vi "DMARS_Frame_v2_write_PXI.vi"(11 "DMARS":dbl[](array[numeric])) -> (0 "No DMARS string":bool, 3 "string_Out":string)   [LabVIEW 2017]
panel:
  out "unsigned 32bit integer":u32
  out "SubFrame":u8
  out "sec":dbl
  out "size(s)":i32
  out "output array":u8[](array[numeric]) format="%x"
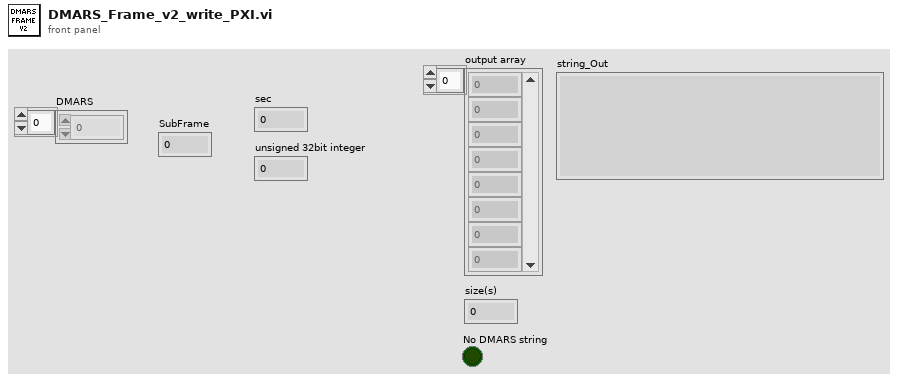
[diagram p1: front panel]
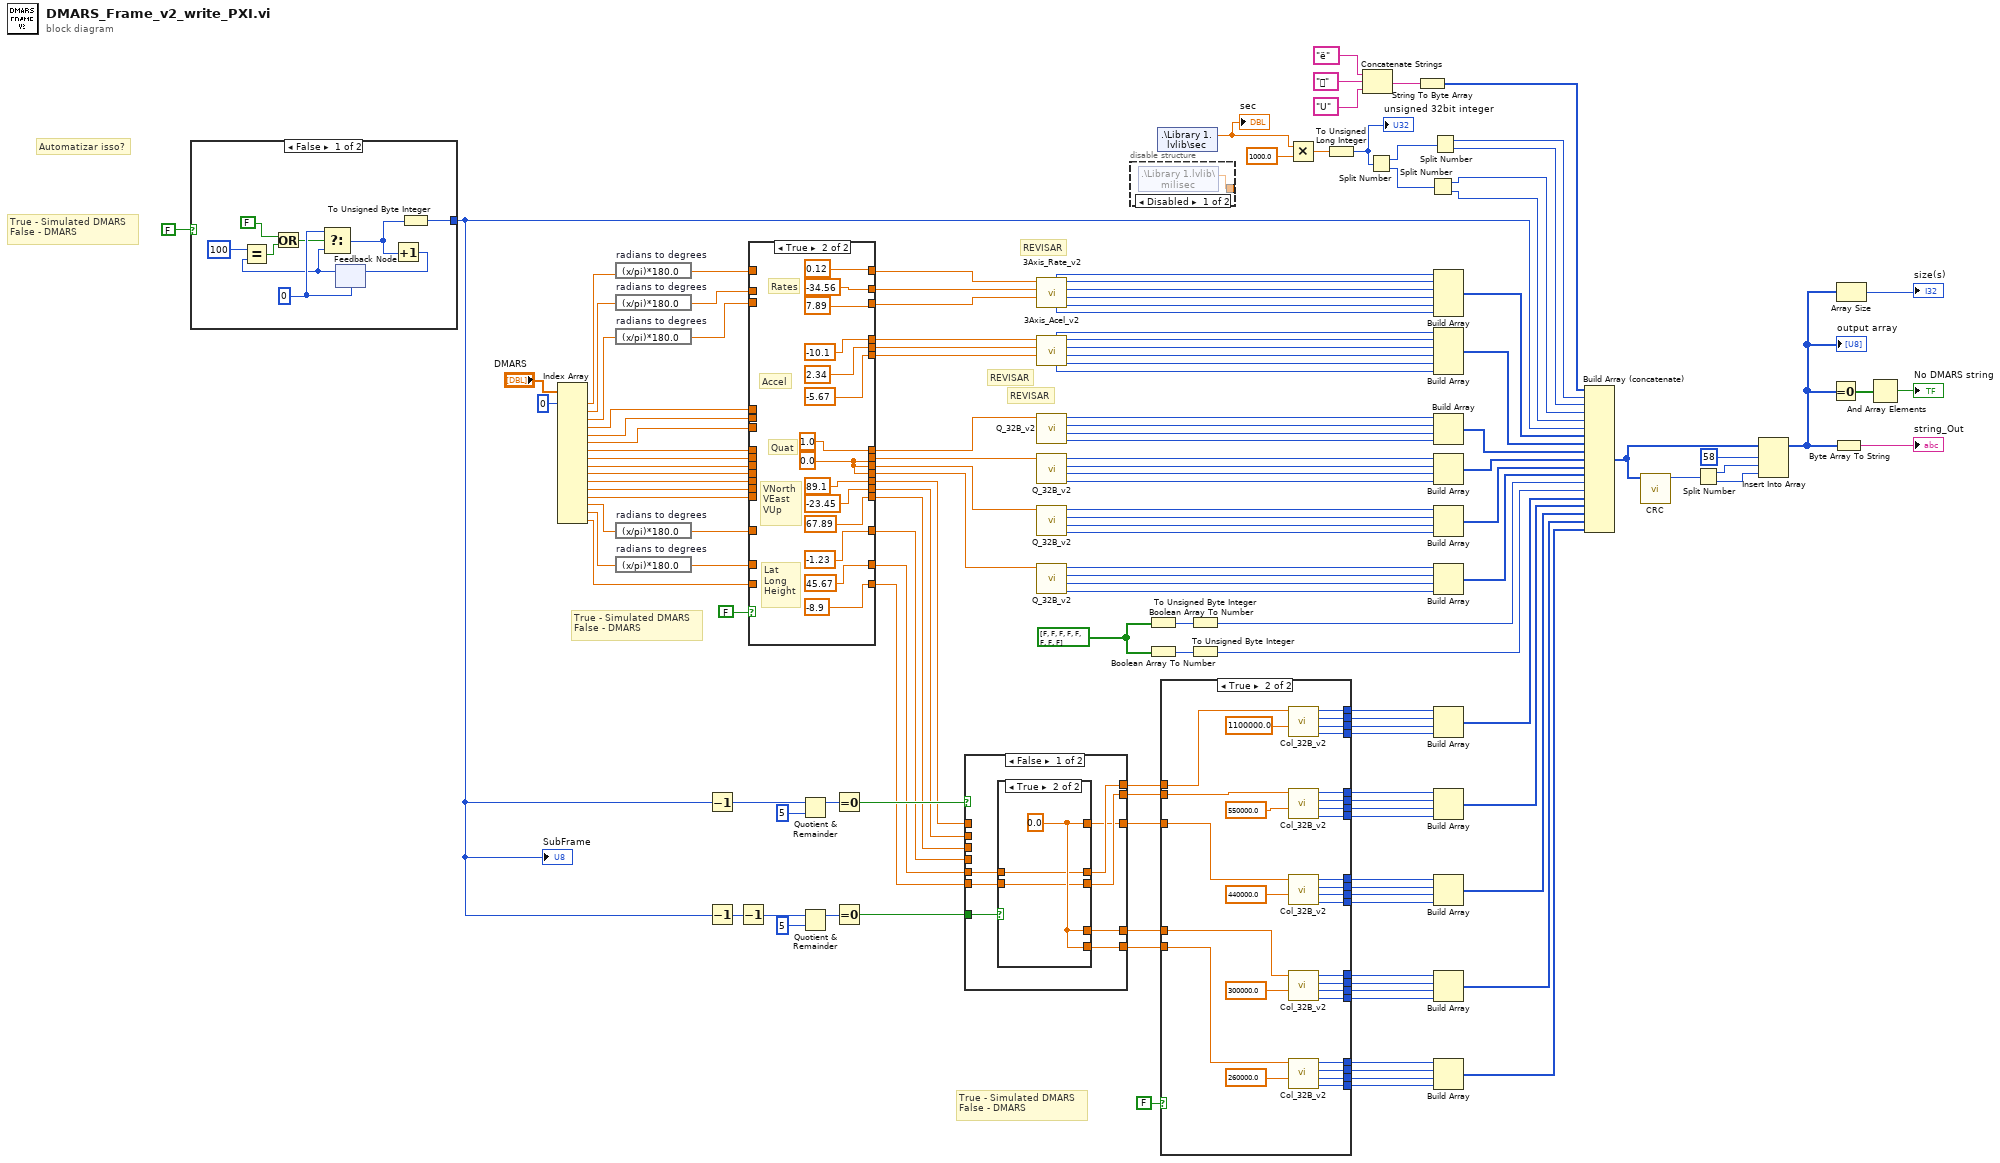
[diagram p0: block diagram]
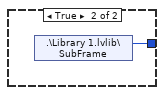
[diagram p2: hidden frame]
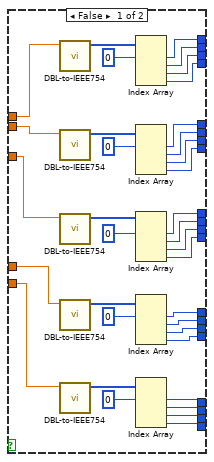
[diagram p5: hidden frame]
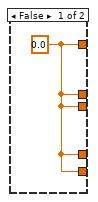
[diagram p6: hidden frame]
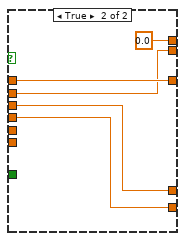
[diagram p7: hidden frame]
diagram:
  w130 = bool[] [FALSE, FALSE, FALSE, FALSE, FALSE, FALSE, FALSE, FALSE] ("Byte 36")
  # "REVISAR"
  # "REVISAR"
  # "REVISAR"
  # "True - Simulated DMARS\nFalse - DMARS"
  # "True - Simulated DMARS\nFalse - DMARS"
  # "Automatizar isso?"
  # "True - Simulated DMARS\nFalse - DMARS"
  n1 = case shown="False" FALSE {
    tunnel: [w148 w156] -> w120
    frame False {
      w155 = 0 ("x")
      n2 = feedback #1(w155) -> (w150:i32)
      n3 = Equal?(x=100, y=w150) -> (x = y?=w151:bool)
      n4 = Or(x=FALSE, y=w151) -> (x .or. y?=w152:bool)
      n5 = Select(t=w155, s=w152, f=w150) -> (s? t:f=w153:i32)
      n6 = Increment(x=w153) -> (x+1=w154:i32)
      n7 = feedback-in #1(w154) -> ()
      n8 = To Unsigned Byte Integer(number=w153) -> (unsigned 8bit integer=w148:u8)
    }
    frame True {
      n9 = shared-variable ".\\Library 1.lvlib\\SubFrame"() -> (w156:u8)  [unwired: 1 in, 1 out]
    }
  }
  "SubFrame" <- w120
  n10 = Index Array(array="DMARS", index #1=0 ("index")) -> (element #1=w79:dbl, element #2=w77:dbl, element #3=w76:dbl, element #4=w105:dbl, element #5=w103:dbl, element #6=w101:dbl, element #7=w99:dbl, element #8=w97:dbl, element #9=w96:dbl, element #10=w93:dbl, element #11=w91:dbl, element #12=w89:dbl, element #13=w87:dbl, element #14=w113:dbl, element #15=w112:dbl, element #16=w81:dbl)  [unwired: 15 in]
  n11 = expression code="(x/pi)*180.0" "radians to degrees"(w79) -> (w78:dbl)
  n12 = expression code="(x/pi)*180.0" "radians to degrees"(w77) -> (w75:dbl)
  n13 = expression code="(x/pi)*180.0" "radians to degrees"(w76) -> (w74:dbl)
  n14 = expression code="(x/pi)*180.0" "radians to degrees"(w113) -> (w85:dbl)
  n15 = expression code="(x/pi)*180.0" "radians to degrees"(w112) -> (w83:dbl)
  n16 = Decrement(x=w120) -> (x-1=w125:u8)
  n17 = Decrement(x=w120) -> (x-1=w121:u8)
  n18 = Decrement(x=w121) -> (x-1=w124:u8)
  n19 = case shown="True" FALSE {
    tunnel: [w172 0.12 ("Numeric")] -> w109
    tunnel: w78 -> [w172 _]
    tunnel: [w171 -34.56 ("Numeric")] -> w108
    tunnel: w75 -> [w171 _]
    tunnel: [w157 7.89 ("Numeric")] -> w107
    tunnel: w74 -> [w157 _]
    tunnel: [w170 -10.1 ("Numeric")] -> w106
    tunnel: w105 -> [w170 _]
    tunnel: [w169 2.34 ("Numeric")] -> w104
    tunnel: w103 -> [w169 _]
    tunnel: [w168 -5.67 ("Numeric")] -> w102
    tunnel: w101 -> [w168 _]
    tunnel: [w167 1.0 ("Numeric")] -> w100
    tunnel: w99 -> [w167 _]
    tunnel: [w166 w179] -> w98
    tunnel: w97 -> [w166 _]
    tunnel: w96 -> [w165 _]
    tunnel: [w165 w179] -> w95
    tunnel: [w164 w179] -> w94
    tunnel: w93 -> [w164 _]
    tunnel: [w163 89.1 ("Numeric")] -> w92
    tunnel: w91 -> [w163 _]
    tunnel: [w162 -23.45 ("Numeric")] -> w90
    tunnel: w89 -> [w162 _]
    tunnel: [w161 67.89 ("Numeric")] -> w88
    tunnel: w87 -> [w161 _]
    tunnel: [w160 -1.23 ("Numeric")] -> w86
    tunnel: w85 -> [w160 _]
    tunnel: [w159 45.67 ("Numeric")] -> w84
    tunnel: w83 -> [w159 _]
    tunnel: [w158 -8.9 ("Numeric")] -> w82
    tunnel: w81 -> [w158 _]
    frame False {
    }
    frame True {
      w179 = 0.0 ("Numeric")
      # "Rates"
      # "Accel"
      # "Quat"
      # "VNorth\nVEast\nVUp"
      # "Lat\nLong\nHeight"
    }
  }
  n20 = Quotient & Remainder(x=w125, y=u8 5) -> (x-y*floor(x/y)=w127:u8)  [unwired: 1 out]
  n21 = Quotient & Remainder(x=w124, y=u8 5) -> (x-y*floor(x/y)=w123:u8)  [unwired: 1 out]
  n22 = Equal To 0?(x=w127) -> (x = 0?=w126:bool)
  n23 = Equal To 0?(x=w123) -> (x = 0?=w114:bool)
  n24 = case shown="False" w126 {
    tunnel: w92 -> [_ w202]
    tunnel: w90 -> [_ w201]
    tunnel: w88 -> [_ w200]
    tunnel: w86 -> [_ w199]
    tunnel: [w191 0.0] -> w119
    tunnel: [w189 w202] -> w118
    tunnel: [w190 w201] -> w117
    tunnel: [w188 w200] -> w116
    tunnel: [w187 w199] -> w115
    tunnel: w114 -> [w194 _]
    tunnel: w84 -> [w193 _]
    tunnel: w82 -> [w192 _]
    frame False {
      n25 = case shown="True" w194 {
        tunnel: w193 -> [_ w197]
        tunnel: w192 -> [_ w196]
        tunnel: [w195 w197] -> w191
        tunnel: [w195 w196] -> w190
        tunnel: [w195 w198] -> w189
        tunnel: [w195 w198] -> w188
        tunnel: [w195 w198] -> w187
        frame False {
          w195 = 0.0
        }
        frame True {
          w198 = 0.0
        }
      }
    }
    frame True {
    }
  }
  n26 = call "3Axis_Rate_v2.vi"("Roll_R"=w107, "Yaw_R"=w108, "Pitch_R"=w109) -> ("RRH"=w57:u8, "YRL"=w58:u8, "YRH"=w59:u8, "PRL"=w60:u8, "RRL"=w56:u8, "PRH"=w61:u8)  [unwired: 3 in]
  n27 = call "3Axis_Acel_v2.vi"("Roll_A"=w102, "Yaw_A"=w104, "Pitch_A"=w106) -> ("RAH"=w50:u8, "YAL"=w51:u8, "YAH"=w52:u8, "PAL"=w53:u8, "RAL"=w49:u8, "PAH"=w54:u8)  [unwired: 3 in]
  n28 = call "Q_32B_v2.vi"("Q_32B"=w100) -> ("LL"=w44:u8, "HL"=w45:u8, "LH"=w46:u8, "HH"=w47:u8)  [unwired: 7 in]
  n29 = call "Q_32B_v2.vi"("Q_32B"=w98) -> ("LL"=w39:u8, "HL"=w40:u8, "LH"=w41:u8, "HH"=w42:u8)  [unwired: 7 in]
  n30 = call "Q_32B_v2.vi"("Q_32B"=w95) -> ("LL"=w34:u8, "HL"=w35:u8, "LH"=w36:u8, "HH"=w37:u8)  [unwired: 7 in]
  n31 = call "Q_32B_v2.vi"("Q_32B"=w94) -> ("LL"=w29:u8, "HL"=w30:u8, "LH"=w31:u8, "HH"=w32:u8)  [unwired: 7 in]
  n32 = disable-structure shown="Disabled" {
    disable-tunnel: [w204 _] -> _
    frame Disabled {
      n33 = shared-variable ".\\Library 1.lvlib\\milisec"() -> (w204:dbl)  [unwired: 1 in, 1 out]
    }
    frame Enabled {
    }
  }
  n34 = Boolean Array To Number(Boolean array=w130) -> (number=w140:u32)
  n35 = Boolean Array To Number(Boolean array=w130) -> (number=w139:u32)
  n36 = shared-variable ".\\Library 1.lvlib\\sec"() -> (w63:dbl)  [unwired: 1 in, 1 out]
  "sec" <- w63
  n37 = case shown="True" FALSE {
    tunnel: [w208 w269] -> w5
    tunnel: [w205 w268] -> w2
    tunnel: [w206 w267] -> w3
    tunnel: [w207 w266] -> w4
    tunnel: [w209 w265] -> w7
    tunnel: [w210 w264] -> w8
    tunnel: [w211 w263] -> w9
    tunnel: [w212 w262] -> w10
    tunnel: [w217 w261] -> w12
    tunnel: [w218 w260] -> w13
    tunnel: [w219 w259] -> w14
    tunnel: [w220 w258] -> w15
    tunnel: [w223 w257] -> w17
    tunnel: [w224 w256] -> w18
    tunnel: [w225 w255] -> w19
    tunnel: [w226 w254] -> w20
    tunnel: [w230 w253] -> w22
    tunnel: [w231 w252] -> w23
    tunnel: [w232 w251] -> w24
    tunnel: [w233 w250] -> w25
    tunnel: w119 -> [w239 w249]
    tunnel: w118 -> [w237 w248]
    tunnel: w117 -> [w238 w247]
    tunnel: w116 -> [w236 w246]
    tunnel: w115 -> [w235 w245]
    frame False {
      n38 = call "DBL-to-IEEE754.vi"("Input_DBL"=w239) -> ("Output_U8"=w234:u8[])  [unwired: 10 in]
      n39 = call "DBL-to-IEEE754.vi"("Input_DBL"=w238) -> ("Output_U8"=w228:u8[])  [unwired: 10 in]
      n40 = call "DBL-to-IEEE754.vi"("Input_DBL"=w237) -> ("Output_U8"=w221:u8[])  [unwired: 10 in]
      n41 = call "DBL-to-IEEE754.vi"("Input_DBL"=w236) -> ("Output_U8"=w213:u8[])  [unwired: 10 in]
      n42 = call "DBL-to-IEEE754.vi"("Input_DBL"=w235) -> ("Output_U8"=w214:u8[])  [unwired: 10 in]
      n43 = Index Array(array=w234, index #1=0 ("index")) -> (element #1=w233:u8, element #2=w232:u8, element #3=w231:u8, element #4=w230:u8)  [unwired: 3 in]
      n44 = Index Array(array=w228, index #1=0 ("index")) -> (element #1=w226:u8, element #2=w225:u8, element #3=w224:u8, element #4=w223:u8)  [unwired: 3 in]
      n45 = Index Array(array=w221, index #1=0 ("index")) -> (element #1=w220:u8, element #2=w219:u8, element #3=w218:u8, element #4=w217:u8)  [unwired: 3 in]
      n46 = Index Array(array=w213, index #1=0 ("index")) -> (element #1=w212:u8, element #2=w211:u8, element #3=w210:u8, element #4=w209:u8)  [unwired: 3 in]
      n47 = Index Array(array=w214, index #1=0 ("index")) -> (element #1=w208:u8, element #2=w207:u8, element #3=w206:u8, element #4=w205:u8)  [unwired: 3 in]
    }
    frame True {
      n48 = call "Col_32B_v2.vi"("Ref"=1100000.0, "Col"=w249) -> ("LL"=w253:u8, "LH"=w252:u8, "HL"=w251:u8, "HH"=w250:u8)  [unwired: 6 in]
      n49 = call "Col_32B_v2.vi"("Ref"=550000.0, "Col"=w247) -> ("LL"=w257:u8, "LH"=w256:u8, "HL"=w255:u8, "HH"=w254:u8)  [unwired: 6 in]
      n50 = call "Col_32B_v2.vi"("Ref"=440000.0, "Col"=w248) -> ("LL"=w261:u8, "LH"=w260:u8, "HL"=w259:u8, "HH"=w258:u8)  [unwired: 6 in]
      n51 = call "Col_32B_v2.vi"("Ref"=300000.0, "Col"=w246) -> ("LL"=w265:u8, "LH"=w264:u8, "HL"=w263:u8, "HH"=w262:u8)  [unwired: 6 in]
      n52 = call "Col_32B_v2.vi"("Ref"=260000.0, "Col"=w245) -> ("LL"=w268:u8, "LH"=w267:u8, "HL"=w266:u8, "HH"=w269:u8)  [unwired: 6 in]
    }
  }
  n53 = To Unsigned Byte Integer(number=w140) -> (unsigned 8bit integer=w27:u8)
  n54 = To Unsigned Byte Integer(number=w139) -> (unsigned 8bit integer=w26:u8)
  n55 = Multiply(x=w63, y=1000.0) -> (x*y=w64:dbl)
  n56 = To Unsigned Long Integer(number=w64) -> (unsigned 32bit integer=w68:u32)
  "unsigned 32bit integer" <- w68
  n57 = Concatenate Strings("ë", "", "U") -> (w135:string)
  n58 = Split Number(x=w68) -> (hi(x)=w67:u16, lo(x)=w66:u16)
  n59 = String To Byte Array(string=w135) -> (unsigned byte array=w141:u8[])
  n60 = Split Number(x=w66) -> (hi(x)=w143:u8, lo(x)=w144:u8)
  n61 = Split Number(x=w67) -> (hi(x)=w145:u8, lo(x)=w146:u8)
  n62 = Build Array(w61, w60, w59, w58, w57, w56) -> (w55:u8[])
  n63 = Build Array(w54, w53, w52, w51, w50, w49) -> (w48:u8[])
  n64 = Build Array(w47, w46, w45, w44) -> (w43:u8[])
  n65 = Build Array(w42, w41, w40, w39) -> (w38:u8[])
  n66 = Build Array(w37, w36, w35, w34) -> (w33:u8[])
  n67 = Build Array(w32, w31, w30, w29) -> (w28:u8[])
  n68 = Build Array(w25, w24, w23, w22) -> (w21:u8[])
  n69 = Build Array(w20, w19, w18, w17) -> (w16:u8[])
  n70 = Build Array(w15, w14, w13, w12) -> (w11:u8[])
  n71 = Build Array(w10, w9, w8, w7) -> (w6:u8[])
  n72 = Build Array(w5, w4, w3, w2) -> (w1:u8[])
  n73 = Build Array (concatenate)(w141, w145, w146, w143, w144, w120, w55, w48, w43, w38, w33, w28, w27, w26, w21, w16, w11, w6, w1) -> (w70:u8[])
  n74 = call "CRC.vi"("Array"=w70) -> ("CRC"=w69:u16)  [unwired: 10 in]
  n75 = Split Number(x=w69) -> (hi(x)=w133:u8, lo(x)=w132:u8)
  n76 = Insert Into Array(array=w70, index=58, new element #1=w133, new element #2=w132) -> (w73:u8[])
  "output array" <- w73
  n77 = Equal To 0?(x=w73) -> (x = 0?=w72:bool[])
  n78 = Byte Array To String(unsigned byte array=w73) -> (string=→"string_Out":string)
  n79 = Array Size(array=w73) -> (size(s)=→"size(s)":i32)
  n80 = And Array Elements(Boolean array=w72) -> (logical AND=→"No DMARS string":bool)
